vi "Introspection Core.vi"(8 "error in (no error)":errorcluster, 11 "CS++DMM in":refnum<class "CS++DMM.lvclass">) -> (0 "error out":errorcluster, 2 "CS++Messages":refnum<class "Message.lvclass">[](array[class]), 3 "CS++DMM out":refnum<class "CS++DMM.lvclass">)   [LabVIEW 2014, in "CS++DMM.lvlib" / "CS++DMM.lvclass"]
doc: "This vi delivers a list with all messages this actor reacts to. \n\nNote that all inherited classes have to overwrite it."
uses:
  CS++DMM.lvclass
  <vilib>/ActorFramework/Message/Message.lvclass
  CS++DMM Messages/Configure Meas Complete Dest [MP] Msg/Configure Meas Complete Dest [MP] Msg.lvclass
  CS++DMM Messages/Configure Multi-Point [MP] Msg/Configure Multi-Point [MP] Msg.lvclass
  CS++DMM Messages/Configure Auto Zero Mode [AZ] Msg/Configure Auto Zero Mode [AZ] Msg.lvclass
  CS++DMM Messages/Configure Power Line Frequency [PLF] Msg/Configure Power Line Frequency [PLF] Msg.lvclass
  CS++DMM Messages/Configure Tranducer Type [TMP] Msg/Configure Tranducer Type [TMP] Msg.lvclass
  CS++DMM Messages/Configure Thermocouple [TC] Msg/Configure Thermocouple [TC] Msg.lvclass
  CS++DMM Messages/Configure Fixed Ref Junction [TC] Msg/Configure Fixed Ref Junction [TC] Msg.lvclass
  CS++DMM Messages/Configure RTD [RTD] Msg/Configure RTD [RTD] Msg.lvclass
  CS++DMM Messages/Configure Thermistor [THM] Msg/Configure Thermistor [THM] Msg.lvclass
  CS++DMM Messages/Configure AC Bandwidth [AC] Msg/Configure AC Bandwidth [AC] Msg.lvclass
  CS++DMM Messages/Configure Frequency Voltage Range [FVR] Msg/Configure Frequency Voltage Range [FVR] Msg.lvclass
  CS++DMM Messages/Configure Trigger Msg/Configure Trigger Msg.lvclass
  CS++DMM Messages/Configure Trigger Slope [TS] Msg/Configure Trigger Slope [TS] Msg.lvclass
  CS++DMM Messages/Configure Measurement Msg/Configure Measurement Msg.lvclass
  CS++DMM Messages/Abort Msg/Abort Msg.lvclass
  CS++DMM Messages/Fetch Msg/Fetch Msg.lvclass
  CS++DMM Messages/Fetch Multi-Point [MP] Msg/Fetch Multi-Point [MP] Msg.lvclass
  CS++DMM Messages/Initiate Msg/Initiate Msg.lvclass
  CS++DMM Messages/Send Software Trigger Msg/Send Software Trigger Msg.lvclass
  CS++DMM Messages/Read Multi-Point [MP] Msg/Read Multi-Point [MP] Msg.lvclass
  CS++DMM Messages/Read Single-Point Msg/Read Single-Point Msg.lvclass
  CSPP_Core/Actors/CS++DeviceActor/CS++DeviceActor.lvclass
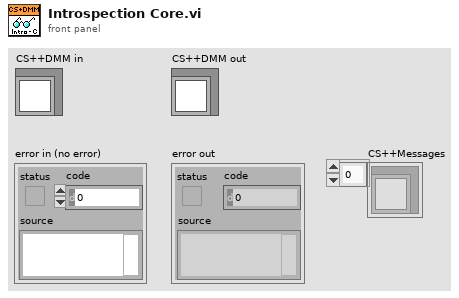
[diagram p1: front panel]
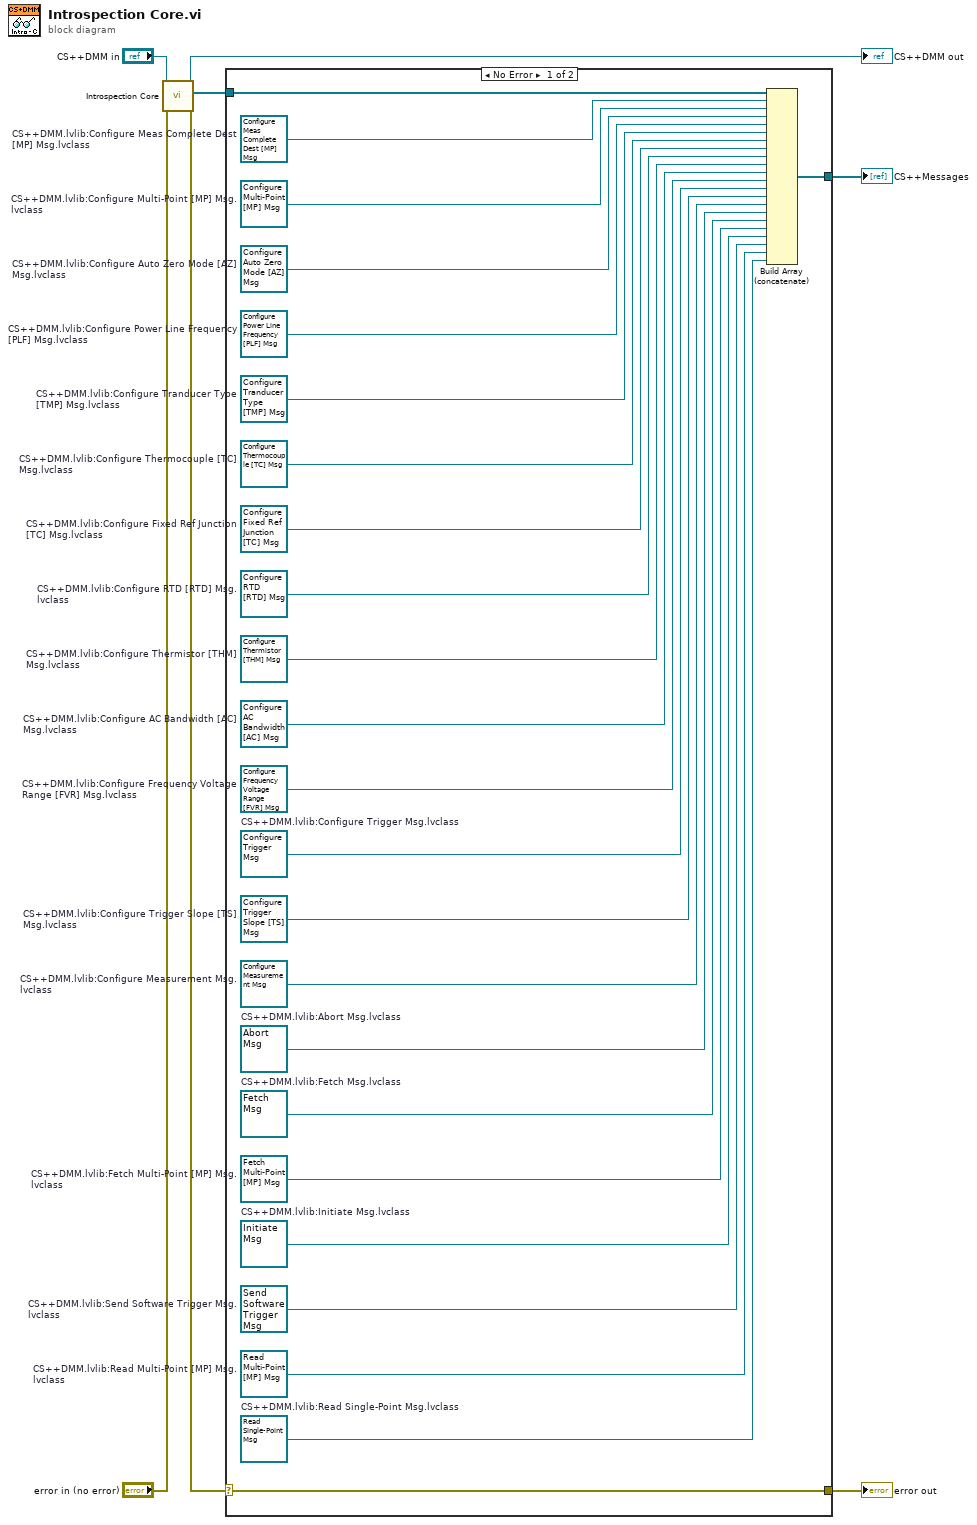
[diagram p0: block diagram]
diagram:
  n1 = call-parent "Introspection Core.vi"("error in (no error)"="error in (no error)", "CS++DeviceActor in"="CS++DMM in") -> ("error out"=w4:errorcluster, "CS++Messages"=w2:refnum<class "Message.lvclass">[], "CS++DeviceActor out"=→"CS++DMM out":refnum<class "CS++DMM.lvclass">)  [unwired: 7 in]
  n2 = case shown="No Error" w4 {
    selector: w4 -> [w31 w32]
    tunnel: [w31 w32] -> w3
    tunnel: w2 -> [w30 _]
    tunnel: [w8 _] -> w1
    frame No Error {
      w9 = refnum<class "Read Single-Point Msg.lvclass"> refnum  # CS++DMM.lvlib:Read Single-Point Msg.lvclass
      w10 = refnum<class "Read Multi-Point [MP] Msg.lvclass"> refnum  # CS++DMM.lvlib:Read Multi-Point [MP] Msg.lvclass
      w11 = refnum<class "Send Software Trigger Msg.lvclass"> refnum  # CS++DMM.lvlib:Send Software Trigger Msg.lvclass
      w12 = refnum<class "Initiate Msg.lvclass"> refnum  # CS++DMM.lvlib:Initiate Msg.lvclass
      w13 = refnum<class "Fetch Multi-Point [MP] Msg.lvclass"> refnum  # CS++DMM.lvlib:Fetch Multi-Point [MP] Msg.lvclass
      w14 = refnum<class "Fetch Msg.lvclass"> refnum  # CS++DMM.lvlib:Fetch Msg.lvclass
      w15 = refnum<class "Abort Msg.lvclass"> refnum  # CS++DMM.lvlib:Abort Msg.lvclass
      w16 = refnum<class "Configure Measurement Msg.lvclass"> refnum  # CS++DMM.lvlib:Configure Measurement Msg.lvclass
      w17 = refnum<class "Configure Trigger Slope [TS] Msg.lvclass"> refnum  # CS++DMM.lvlib:Configure Trigger Slope [TS] Msg.lvclass
      w18 = refnum<class "Configure Trigger Msg.lvclass"> refnum  # CS++DMM.lvlib:Configure Trigger Msg.lvclass
      w19 = refnum<class "Configure Frequency Voltage Range [FVR] Msg.lvclass"> refnum  # CS++DMM.lvlib:Configure Frequency Voltage Range [FVR] Msg.lvclass
      w20 = refnum<class "Configure AC Bandwidth [AC] Msg.lvclass"> refnum  # CS++DMM.lvlib:Configure AC Bandwidth [AC] Msg.lvclass
      w21 = refnum<class "Configure Thermistor [THM] Msg.lvclass"> refnum  # CS++DMM.lvlib:Configure Thermistor [THM] Msg.lvclass
      w22 = refnum<class "Configure RTD [RTD] Msg.lvclass"> refnum  # CS++DMM.lvlib:Configure RTD [RTD] Msg.lvclass
      w23 = refnum<class "Configure Fixed Ref Junction [TC] Msg.lvclass"> refnum  # CS++DMM.lvlib:Configure Fixed Ref Junction [TC] Msg.lvclass
      w24 = refnum<class "Configure Thermocouple [TC] Msg.lvclass"> refnum  # CS++DMM.lvlib:Configure Thermocouple [TC] Msg.lvclass
      w25 = refnum<class "Configure Tranducer Type [TMP] Msg.lvclass"> refnum  # CS++DMM.lvlib:Configure Tranducer Type [TMP] Msg.lvclass
      w26 = refnum<class "Configure Power Line Frequency [PLF] Msg.lvclass"> refnum  # CS++DMM.lvlib:Configure Power Line Frequency [PLF] Msg.lvclass
      w27 = refnum<class "Configure Auto Zero Mode [AZ] Msg.lvclass"> refnum  # CS++DMM.lvlib:Configure Auto Zero Mode [AZ] Msg.lvclass
      w28 = refnum<class "Configure Multi-Point [MP] Msg.lvclass"> refnum  # CS++DMM.lvlib:Configure Multi-Point [MP] Msg.lvclass
      w29 = refnum<class "Configure Meas Complete Dest [MP] Msg.lvclass"> refnum  # CS++DMM.lvlib:Configure Meas Complete Dest [MP] Msg.lvclass
      n3 = Build Array (concatenate)(w30, w29, w28, w27, w26, w25, w24, w23, w22, w21, w20, w19, w18, w17, w16, w15, w14, w13, w12, w11, w10, w9) -> (w8:refnum<class "Message.lvclass">[])
    }
    frame Error {
    }
  }
  "error out" <- w3
  "CS++Messages" <- w1
